vi "nanomsg_setsocketopt.vi"(0 "socket in":refnum<class "nanomsg_socket.lvclass">, 1 "option":i32=3, 2 "value":variant, 3 "error in":errorcluster, 4 "level":i32=3) -> (5 "socket out":refnum<class "nanomsg_socket.lvclass">, 6 "error out":errorcluster)   [LabVIEW 2014, in "nanomsg.lvlib" / "nanomsg_socket.lvclass"]
doc: "Sets the specified <b>option</b> to the given <b>value</b>. The type of data connected to value must match that expected by the option (see the API documentation).\n\nNote that LabVIEW strings are used for \"raw\" data.\n\nDetailed API documentation: http://nanomsg.org/documentation.html"
uses:
  nanomsg_socket.lvclass
  nanomsg_socket.lvclass/nanomsg_socket.ctl
  <vilib>/Utility/error.llb/Error Cluster From Error Code.vi
  nanomsg.lvlib
panel:
  out "option code":i32
  # "NN"
  # "labview"
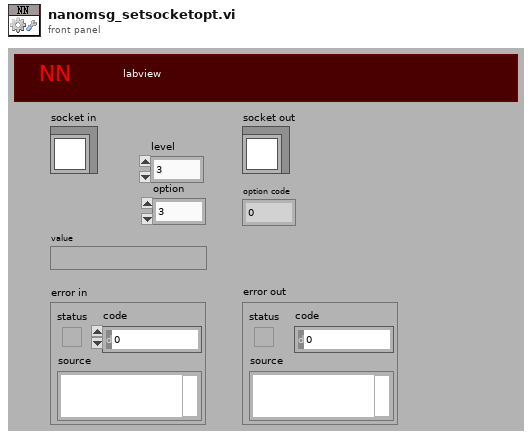
[diagram p1: front panel]
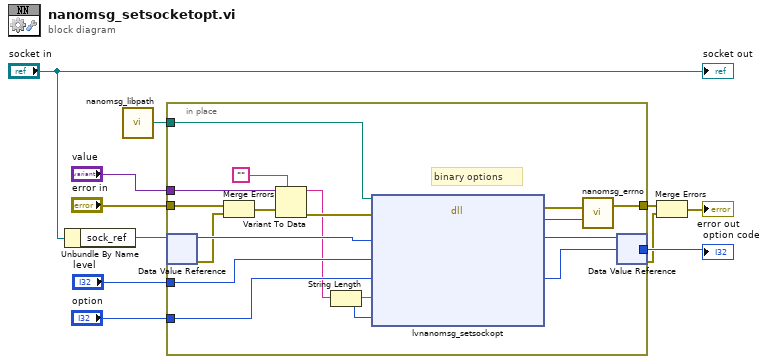
[diagram p0: block diagram]
diagram:
  n1 = Unbundle By Name("socket in") -> ("sock_ref"=w5:refnum<data-value>)
  n2 = call "nanomsg_libpath.vi"() -> ("path"=w4:path)
  n3 = in-place {
    in-place-border: [w26] -> w11
    in-place-border: "value" -> [w25]
    in-place-border: "error in" -> [w24]
    in-place-border: "option" -> [w23]
    in-place-border: [w22] -> w7
    in-place-border: w4 -> [w19]
    in-place-border: "level" -> [w16]
    # "binary options"
    n4 = in-place-dvr #1(w5) -> (w21:u64, w17:errorcluster)
    n5 = Merge Errors(w24, w17) -> (w18:errorcluster)
    n6 = Variant To Data(error in=w18, type="", Variant=w25) -> (data=w12:string, error out=w14:errorcluster)
    n7 = String Length(string=w12) -> (length=w13:i32)
    n8 = dll-call lib="?" fn="lvnanomsg_setsockopt" ("zmq_labview.dll:lvzmq_setsockopt")(path in=w19, error in=w14, "socket"=w21, "level"=w16, "option"=w23, "data"=w12, "len"=w13) -> (error out=w28:errorcluster, "return type"=w27:i32, "socket"=w20:u64, "option"=w22:i32)  [unwired: 4 in, 1 out]
    n9 = call "nanomsg_errno.vi"("retval"=w27, "error in"=w28) -> ("error out"=w26:errorcluster)  [unwired: 1 out]
    n10 = in-place-dvr #1(w20) -> (w2:errorcluster)  [unwired: 1 out]
  }
  "option code" <- w7
  n11 = Merge Errors(w11, w2) -> (→"error out":errorcluster)
  "socket out" <- "socket in"
